vi "Strip Blank Strings.vi"(11 "ArrayIn":string[](array[string])) -> (3 "Array Out":string[](array[string]))   [LabVIEW 2023]
doc: "This VI takes an array of strings and removes array values with blank entries. This includes any combination of spaces, new line, carraige return, and tab characters. The resulting array is returns in the same order sans removed items"
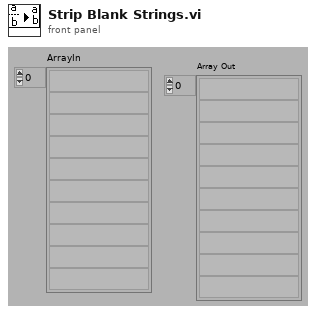
[diagram p1: front panel]
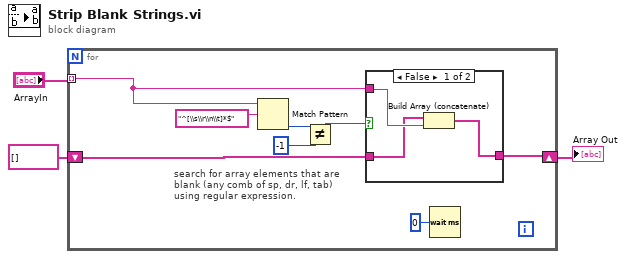
[diagram p0: block diagram]
diagram:
  n1 = for {
    shift-right: [w10] -> w2
    shift-left: string[] [] -> [w11]
    tunnel: "ArrayIn" -> [w5] mode=indexing
    # "search for array elements that are\nblank (any comb of sp, dr, lf, tab) \nusing regular expression."
    n2 = Match Pattern(string=w5, regular expression="^[\\s\\r\\n\\t]*$") -> (offset past match=w8:i32)  [unwired: 1 in, 3 out]
    n3 = Not Equal?(x=w8, y=-1) -> (x != y?=w6:bool)
    n4 = case shown="False" w6 {
      tunnel: w11 -> [w13 w15]
      tunnel: w5 -> [w14 _]
      tunnel: [w12 w15] -> w10
      frame False {
        n5 = Build Array (concatenate)(w13, w14) -> (w12:string[])
      }
      frame True {
      }
    }
    n6 = Wait (ms)(milliseconds to wait=u32 0) -> ()  [unwired: 1 out]
  }
  "Array Out" <- w2
